vi "ProgressPopup_Update.vi"(8 "error in":errorcluster, 11 "Message":string) -> (0 "error out":errorcluster)   [LabVIEW 2022 SP3, in "hse-ui.lvlib"]
doc: "Closes the modal progress window.\n\n\n\n____\nHAMPEL SOFTWARE ENGINEERING v3.8.0 (2023-12-18 14:41)"
uses:
  hse-ui.lvlib
  ProgressPopup.vi
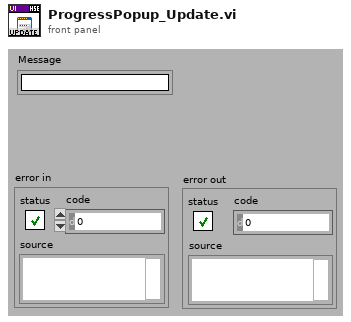
[diagram p1: front panel]
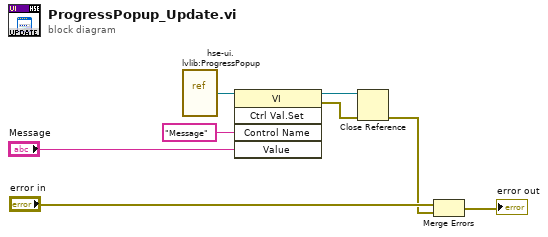
[diagram p0: block diagram]
diagram:
  n1 = vi-ref "hse-ui.lvlib:ProgressPopup.vi"() -> (w4:refnum<vi>)
  n2 = invoke class="VI" method="Ctrl Val.Set"(reference=w4, "Control Name"="Message", "Value"="Message") -> (reference out=w3:refnum<vi>, error out=w2:errorcluster)  [unwired: 2 in, 3 out]
  n3 = Close Reference(reference=w3, error in (no error)=w2) -> (error out=w1:errorcluster)
  n4 = Merge Errors("error in", w1) -> (→"error out":errorcluster)
